vi "cmdElements2Text.vi"(1 "CodeElements":T4={"address"="010000000000", "controlCode"="11", "dataLength"=4.0, "dataSection"="12345678", "checkCode"="7F"}) -> (0 "CommandText":T1)   [LabVIEW 2010]
uses:
  types/OutputDataFormat.ctl
  types/VarableID.ctl
  main/AmmeterGlobalCostants.vi
  Program Files/National Instruments/LabVIEW 2010/resource/objmgr/DOMUserDefRef.rc
panel:
  out "节点类型":i32(ring)=1 items=["Element_Node"=1, "Attribute_Node"=2, "Text_Node"=3, "CDATASection_Node"=4, "EntityReference_Node"=5, "Entity_Node"=6, "ProcessingInstruction_Node"=7, "Comment_Node"=8, "Document_Node"=9, "DocumentType_Node"=10, "DocumentFragment_Node"=11, "Notation_Node"=12]
  out "TextElements":T3
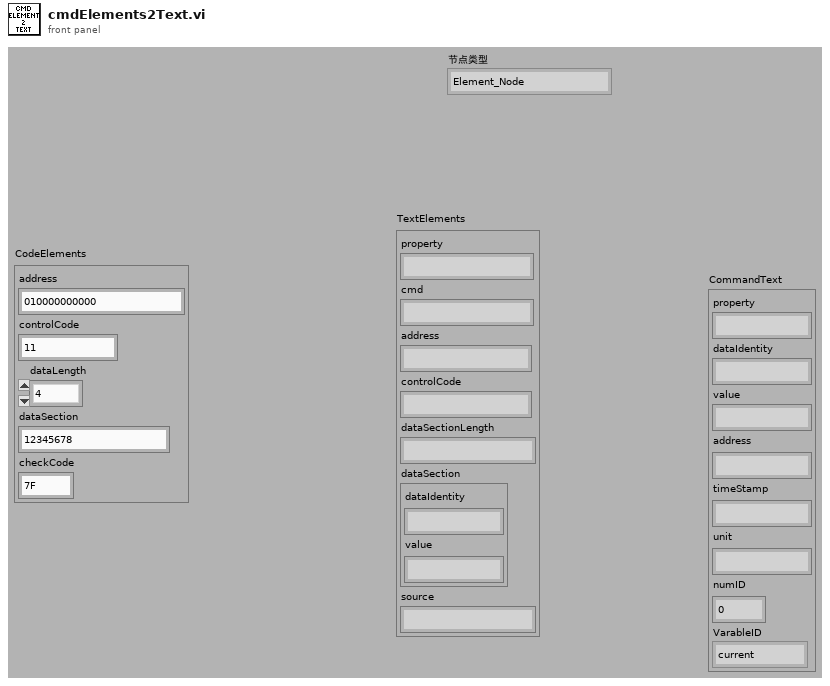
[diagram p1: front panel]
types:
  T1 = typedef "OutputDataFormat.ctl" = cluster{"property":string, "dataIdentity":string, "value":string, "address":string, "timeStamp":string, "unit":string, "numID":i32, "VarableID":T2}
  T2 = typedef "VarableID.ctl" = enum16{"current", "power", "PF", "voltage"}
  T3 = cluster{"property":string, "cmd":string, "address":string, "controlCode":string, "dataSectionLength":string, "dataSection":cluster{"dataIdentity":string, "value":string}, "source":string}
  T4 = cluster{"address":string, "controlCode":string, "dataLength":dbl, "dataSection":string, "checkCode":string}
  T5 = cluster{"property":string, "cmd":string, "address":string, "controlCode":string, "dataSectionLength":string, "dataSection":string, "source":string}
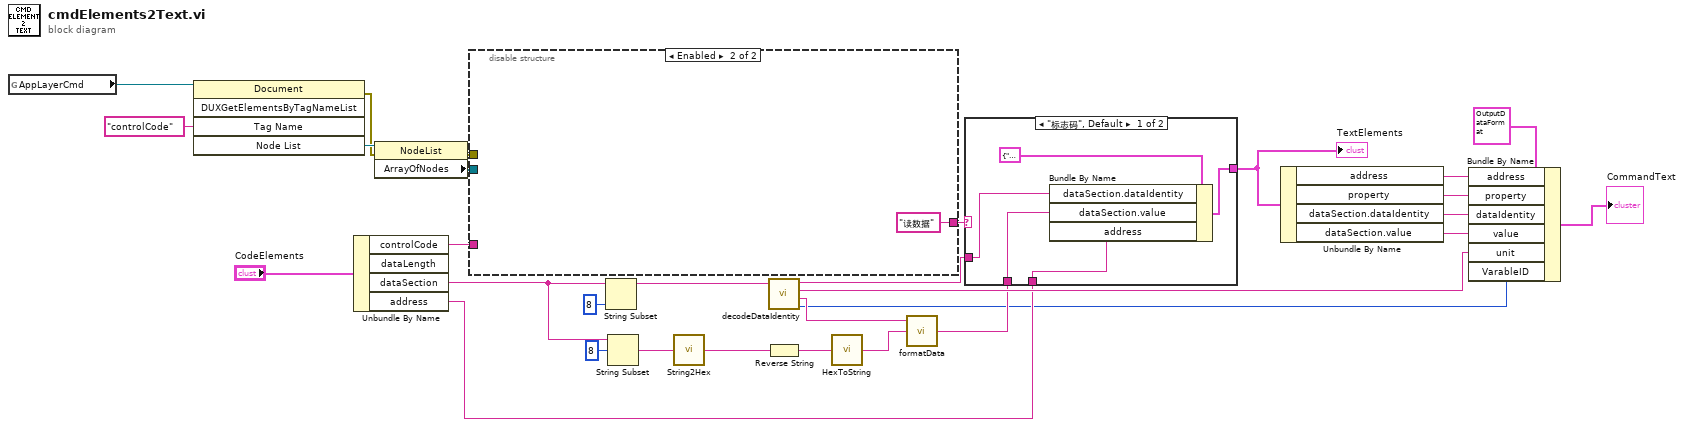
[diagram p0: block diagram]
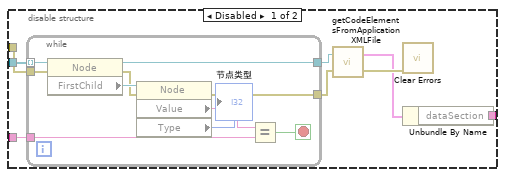
[diagram p2: hidden frame]
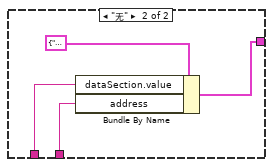
[diagram p3: hidden frame]
diagram:
  n1 = global read "AmmeterGlobalCostants.vi" "AppLayerCmd"() -> (w1:refnum<k20>)
  n2 = invoke class="Document" method="DUXGetElementsByTagNameList"(reference=w1, "Tag Name"="controlCode") -> (error out=w8:errorcluster, "Node List"=w27:refnum<k20>)  [unwired: 3 in, 3 out]
  n3 = Unbundle By Name("CodeElements") -> ("controlCode"=w26:string, "dataSection"=w18:string, "address"=w23:string)  [unwired: 1 out]
  n4 = property class="NodeList"(reference=w27, error in=w8) -> (error out=w7:errorcluster, "ArrayOfNodes"=w25:refnum<k20>[])  [unwired: 1 out]
  n5 = disable-structure shown="Enabled" {
    disable-tunnel: w26 -> [w37 _]
    disable-tunnel: w25 -> [w36 _]
    disable-tunnel: [w33 "读数据" ("dataSection")] -> w24
    disable-tunnel: w7 -> [w32 _]
    frame Disabled {
      n6 = while {
        tunnel: w37 -> [w47]
        tunnel: w36 -> [w48] mode=indexing
        tunnel: [w44] -> w35
        tunnel: w32 -> [w42]
        tunnel: [w40] -> w31
        stop <- w45 stop-if-true
        n7 = property class="Node"(reference=w48, error in=w42) -> (reference out=w44:refnum<k20>, error out=w41:errorcluster, "FirstChild"=w43:refnum<k20>)
        n8 = property class="Node"(reference=w43, error in=w41) -> (error out=w40:errorcluster, "Value"=w46:string, "Type"=→"节点类型":i32)  [unwired: 1 out]
        n9 = Equal?(x=w46, y=w47) -> (x = y?=w45:bool)
      }
      n10 = call "getCodeElementsFromApplicationXMLFile.vi"("error in (no error)"=w31, "Node"=w35) -> ("error out"=w38:errorcluster, "TextElements"=w34:T5)
      n11 = call <vilib>:"Clear Errors.vi"("error in (no error)"=w38) -> ()  [unwired: 6 in, 1 out]
      n12 = Unbundle By Name(w34) -> ("dataSection"=w33:string)
    }
    frame Enabled {
    }
  }
  n13 = String Subset(string=w18, length (rest)=8 ("offset (0)")) -> (substring=w22:string)  [unwired: 1 in]
  n14 = String Subset(string=w18, offset (0)=8) -> (substring=w11:string)  [unwired: 1 in]
  n15 = call "String2Hex.vi"("value"=w11) -> ("String"=w10:string)
  n16 = call "decodeDataIdentity.vi"("dataIdentityCode"=w22) -> ("VarableID"=w3:T2, "dataFormat"=w6:string, "unit"=w30:string, "dataIdentityText"=w2:string)  [unwired: 2 in]
  n17 = Reverse String(1:w10) -> (0:w9:string)
  n18 = call "HexToString.vi"("input Hex"=w9) -> ("output string"=w5:string)
  n19 = call "formatData.vi"("originalData"=w5, "dataFormat"=w6) -> ("formatedData"=w4:string)  [unwired: 2 in, 1 out]
  n20 = case shown="\"标志码\", Default" w24 {
    tunnel: w2 -> [w51 _]
    tunnel: [w54 w57] -> w21
    tunnel: w23 -> [w53 w58]
    tunnel: w4 -> [w50 w55]
    frame "标志码", Default {
      n21 = Bundle By Name(cluster=T3 {"property"="读数据", "cmd"="主站请求帧", "address"="AAAAAAAAAAAA", "controlCode"="11", "dataSectionLength"="04", "dataSection"={"dataIdentity"="", "value"=""}, "source"="主站"} ("TextElements"), "dataSection.dataIdentity"=w51, "dataSection.value"=w50, "address"=w53) -> (w54:T3)
    }
    frame "无" {
      n22 = Bundle By Name(cluster=T3 {"property"="读数据", "cmd"="主站请求帧", "address"="AAAAAAAAAAAA", "controlCode"="11", "dataSectionLength"="04", "dataSection"={"dataIdentity"="", "value"=""}, "source"="主站"} ("TextElements"), "dataSection.value"=w55, "address"=w58) -> (w57:T3)
    }
  }
  "TextElements" <- w21
  n23 = Unbundle By Name(w21) -> ("address"=w12:string, "property"=w17:string, "dataSection.dataIdentity"=w16:string, "dataSection.value"=w15:string)
  n24 = Bundle By Name(cluster=T1 {"property"="", "dataIdentity"="", "value"="", "address"="", "timeStamp"="", "unit"="", "numID"=0, "VarableID"=enum."current"} ("CommandText"), "address"=w12, "property"=w17, "dataIdentity"=w16, "value"=w15, "unit"=w30, "VarableID"=w3) -> (→"CommandText":T1)
